vi "InvokePPP_SystemExe.vi"(8 "error in (no error)":errorcluster, 10 "PPP_parameters":T1, 11 "Py Session":refnum<k35>) -> (0 "error out":errorcluster, 3 "Py Session out":refnum<k35>)   [LabVIEW 2022 SP3, in "DLP2.lvclass"]
uses:
  DLP2.lvclass
  DLP2.lvclass/DLP2.ctl
  TopLevel/Typedefs/PrinterHeads--Enum.ctl
  DataTypes/PPP_Python--cluster.ctl
panel:
  in  "command line":string="perl MyScript.pl argument1"
  out "error out 2":errorcluster
  out "standard error":string
  out "standard output":string
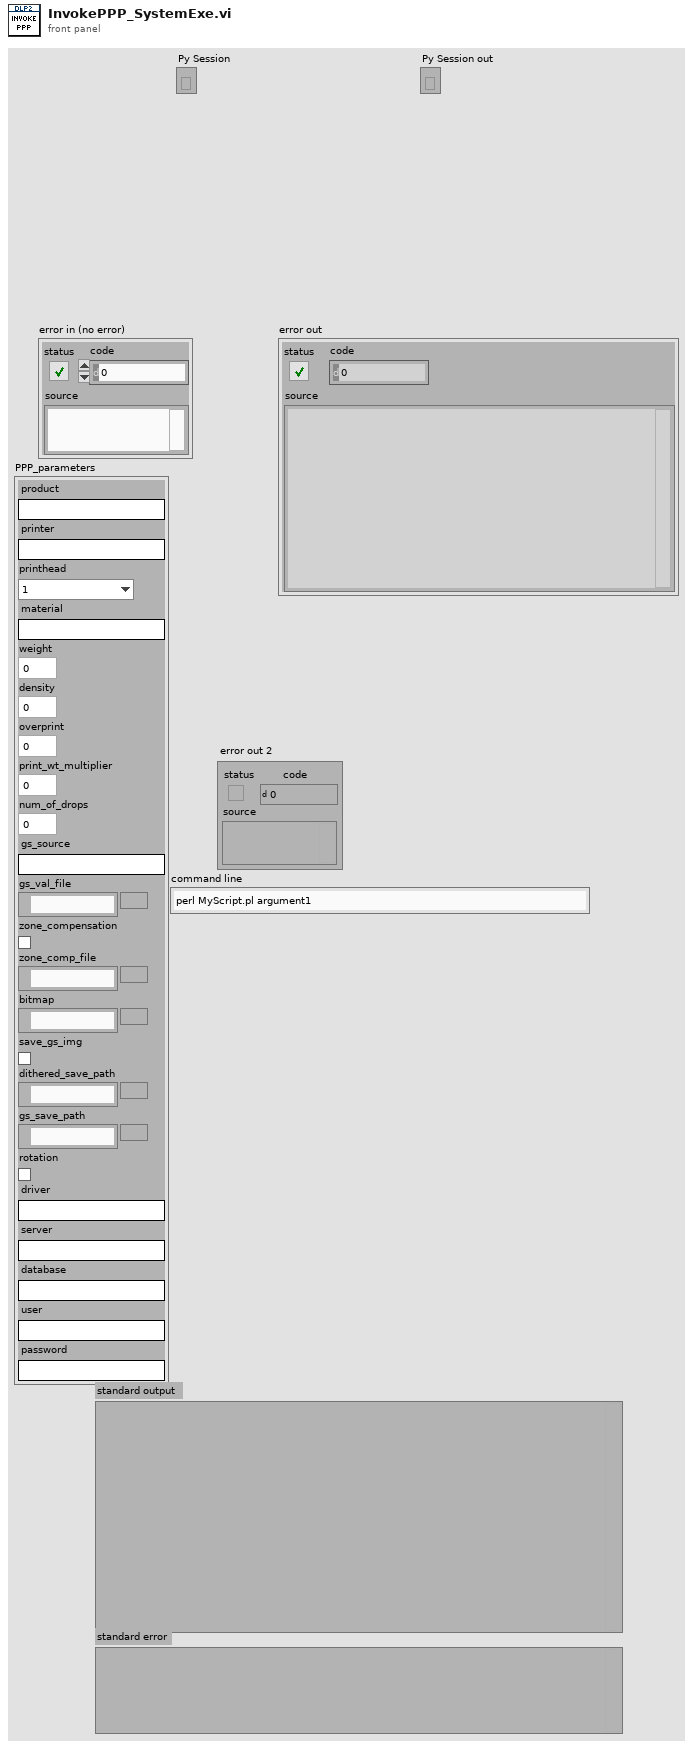
[diagram p1: front panel]
types:
  T1 = typedef "PPP_Python--cluster.ctl" = cluster{"product":string, "printer":string, "printhead":T2, "material":string, "weight":dbl, "density":dbl, "overprint":dbl, "print_wt_multiplier":dbl, "num_of_drops":i32, "gs_source":string, "gs_val_file":path, "zone_compensation":bool, "zone_comp_file":path, "bitmap":path, "save_gs_img":bool, "dithered_save_path":path, "gs_save_path":path, "rotation":bool, "driver":string, "server":string, "database":string, "user":string, "password":string}
  T2 = typedef "PrinterHeads--Enum.ctl" = enum16{"1", "2", "3", "4", "5", "6", "-1"}
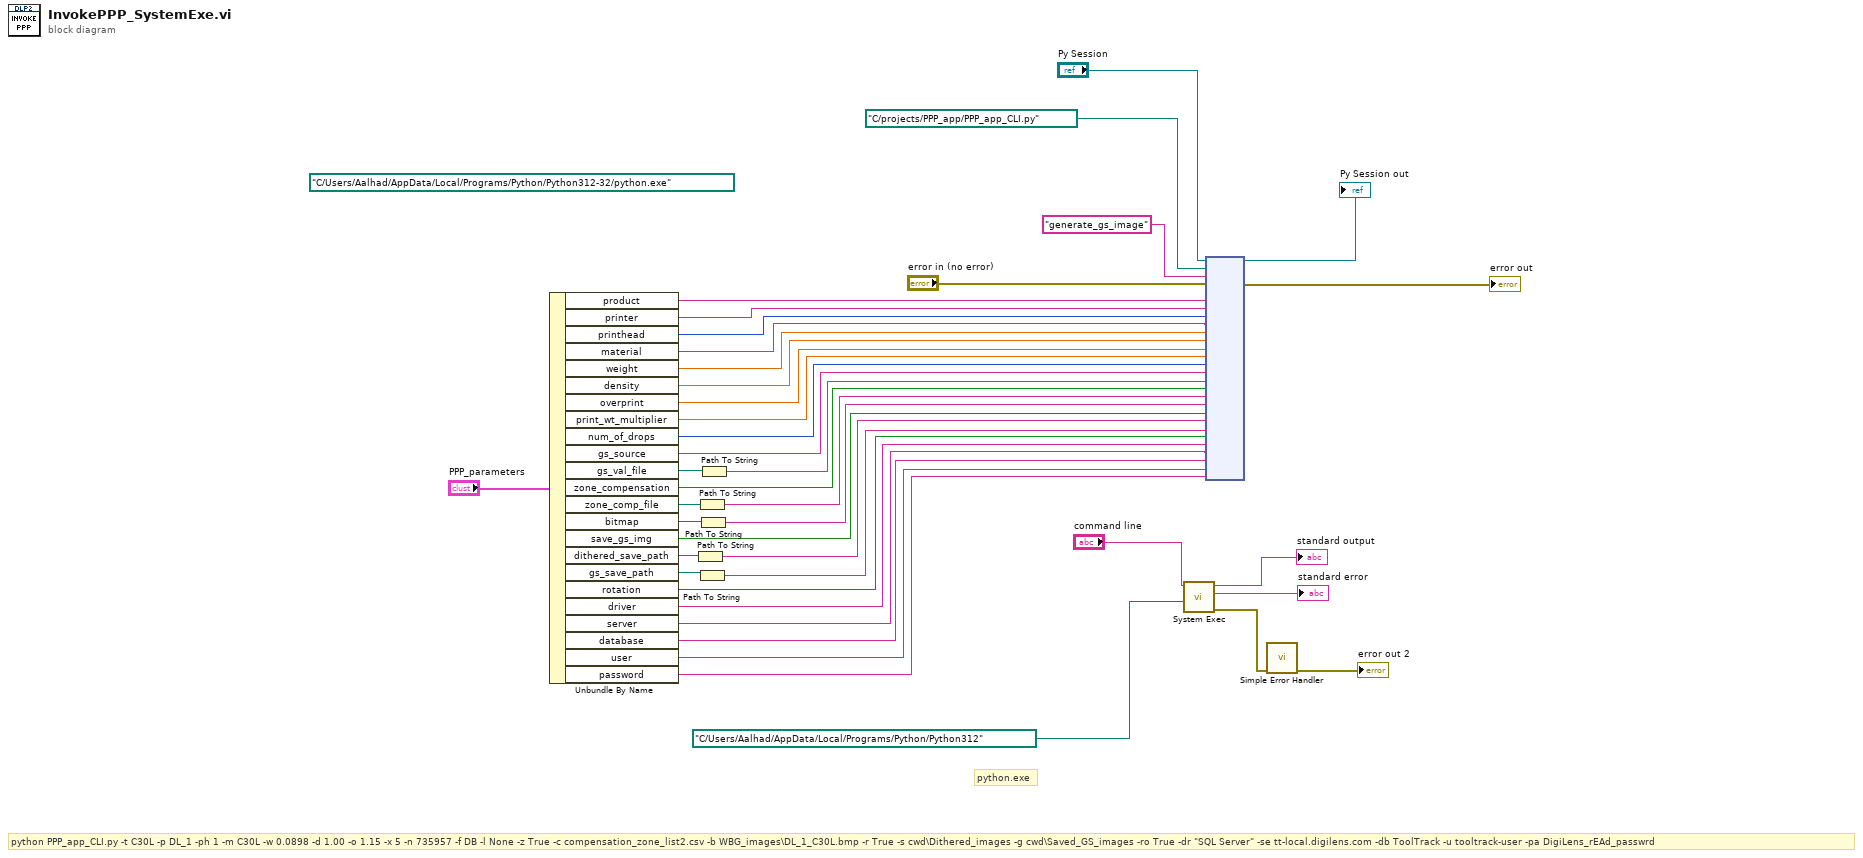
[diagram p0: block diagram]
diagram:
  (unwired) path "C:/Users/Aalhad/AppData/Local/Programs/Python/Python312-32/python.exe" ("Python path")
  # "python PPP_app_CLI.py -t C30L -p DL_1 -ph 1 -m C30L -w 0.0898 -d 1.00 -o 1.15 -x 5 -n 735957 -f DB -l None -z True -c compensation_zone_list2.csv -b WBG_images\\DL_1_C30L.bmp -r True -s cwd\\Dithered_images -g cwd\\Saved_GS_images -ro True -dr \"SQL Server\" -se tt-local.digilens.com -db ToolTrack -u tooltrack-user -pa DigiLens_rEAd_passwrd"
  # "python.exe"
  n1 = Unbundle By Name("PPP_parameters") -> ("product"=w34:string, "printer"=w33:string, "printhead"=w32:T2, "material"=w31:string, "weight"=w30:dbl, "density"=w29:dbl, "overprint"=w28:dbl, "print_wt_multiplier"=w27:dbl, "num_of_drops"=w26:i32, "gs_source"=w25:string, "gs_val_file"=w24:path, "zone_compensation"=w22:bool, "zone_comp_file"=w21:path, "bitmap"=w20:path, "save_gs_img"=w16:bool, "dithered_save_path"=w19:path, "gs_save_path"=w14:path, "rotation"=w12:bool, "driver"=w11:string, "server"=w10:string, "database"=w9:string, "user"=w8:string, "password"=w7:string)
  n2 = Path To String(path=w19) -> (string=w15:string)
  n3 = Path To String(path=w21) -> (string=w18:string)
  n4 = Path To String(path=w14) -> (string=w13:string)
  n5 = Path To String(path=w20) -> (string=w17:string)
  n6 = Path To String(path=w24) -> (string=w23:string)
  n7 = call <vilib>:"System Exec.vi"("working directory"=path "C:/Users/Aalhad/AppData/Local/Programs/Python/Python312" ("Python path"), "command line"="command line") -> ("error out"=w3:errorcluster, "standard error"=→"standard error":string, "standard output"=→"standard output":string)  [unwired: 4 in, 3 out]
  n8 = node("Py Session", path "C:/projects/PPP_app/PPP_app_CLI.py", "generate_gs_image" ("function name"), "error in (no error)", w34, w33, w32, w31, w30, w29, w28, w27, w26, w25, w23, w22, w18, w17, w16, w15, w13, w12, w11, w10, w9, w8, w7) -> (→"Py Session out":refnum<k35>, →"error out":errorcluster)  [unwired: 25 in, 2 out]
  n9 = call <vilib>:"Simple Error Handler.vi"("error in (no error)"=w3) -> ("error out"=→"error out 2":errorcluster)  [unwired: 1 in, 7 out]
